vi "Destroy Events.vi"(8 "error in (no error)":errorcluster, 10 "Events Regs.":refnum<event-registration>, 11 "Events":T1) -> (0 "error out":errorcluster)   [LabVIEW 2017, in "CLI.lvclass"]
uses:
  CLI.lvclass
  Events.ctl
panel:
  # "Connector Pane"
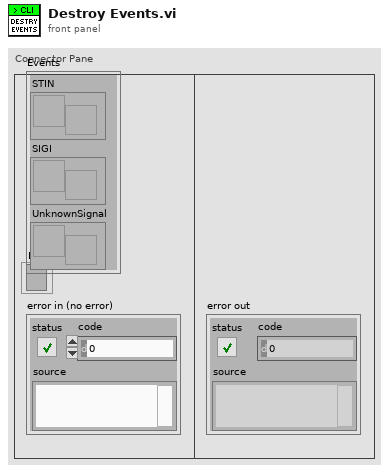
[diagram p1: front panel]
types:
  T1 = typedef "Events.ctl" = cluster{"STIN":refnum<user-event>, "SIGI":refnum<user-event>, "UnknownSignal":refnum<user-event>}
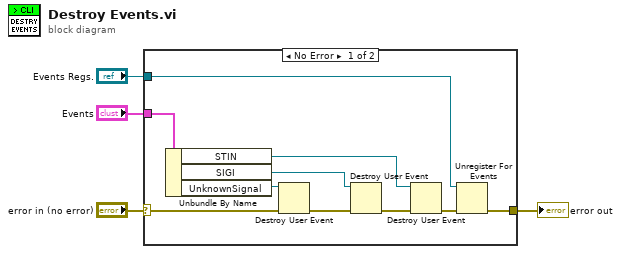
[diagram p0: block diagram]
diagram:
  n1 = case shown="No Error" "error in (no error)" {
    selector: "error in (no error)" -> [w6 w15]
    tunnel: [w13 w15] -> w3
    tunnel: "Events" -> [w14 _]
    tunnel: "Events Regs." -> [w12 _]
    frame No Error {
      n2 = Unbundle By Name(w14) -> ("STIN"=w9:refnum<user-event>, "SIGI"=w8:refnum<user-event>, "UnknownSignal"=w7:refnum<user-event>)
      n3 = Destroy User Event(user event=w7, error in=w6) -> (error out=w5:errorcluster)
      n4 = Destroy User Event(user event=w8, error in=w5) -> (error out=w11:errorcluster)
      n5 = Destroy User Event(user event=w9, error in=w11) -> (error out=w10:errorcluster)
      n6 = Unregister For Events(event registration refnum=w12, error in=w10) -> (error out=w13:errorcluster)
    }
    frame Error {
    }
  }
  "error out" <- w3
